vi "Aero_tunnel_monitor.vi"() -> ()   [LabVIEW 2011]
uses:
  Controls/Post_Process.ctl
  ADAM Client/Sub VIs/ADAM Controls/Update_scan_value.ctl
  Globals/Meas_global.vi
  <userlib>/LV-Link3/PolySubVIs/DtCreateAoutChan.vi
  <userlib>/LV-Link3/PolySubVIs/DtOLWriteSingle.vi
panel:
  in  "Display Graph?":bool
  in  "Menu Ring":u16(ring) items=["Lift", "Pitch", "Drag", "Side", "Yaw", "Roll"]
  in  "Samples":i32=1000
  out "Waveform Chart":dbl[](graph)
  in  "Output Roll":bool
  out "Roll":string="0.0 Nm"
  in  "Output Yaw":bool
  out "Yaw":string="0.0 Nm"
  in  "Output Pitch":bool
  out "Pitch":string="0.0 Nm"
  in  "Output SF":bool
  out "SF":string="0.0 N"
  in  "Output Drag":bool
  out "Drag":string="0.0 N"
  in  "Output Lift":bool
  out "Lift":string="0.0 N"
  in  "Balance Safey limits":T1(array[cluster])=[{"Max +ve Range"=80, "Max -ve Range"=80, "Axis"="Lift"}, {"Max +ve Range"=80, "Max -ve Range"=80, "Axis"="Pitch"}, {"Max +ve Range"=80, "Max -ve Range"=80, "Axis"="Drag"}, {"Max +ve Range"=80, "Max -ve Range"=80, "Axis"="Side-Force"}, {"Max +ve Range"=99, "Max -ve Range"=99, "Axis"="Yaw"}, {"Max +ve Range"=80, "Max -ve Range"=80, "Axis"="Roll"}] {"Max -ve Range" min=0 max=100; "Max +ve Range" min=0 max=100}
  out "Monitor Speed (Hz)":dbl=1765.7669969251795
  out "Belt slip warning":bool
  out "Road Status":string="???"
  in  "GotoYaw":bool
  in  "NewYawPos":dbl
  out "YAW POSITION":dbl
  out "Required WindSpeedRatio":dbl
  out "ROAD SPEED m/s":dbl
  in  "BL Fan1":i32
  in  "BL Fan2":i32
  in  "Stop drive":bool
  in  "Start Drive":bool
  in  "Synch to Wind":bool
  out "Road Info":string="???"
  in  "stop":bool
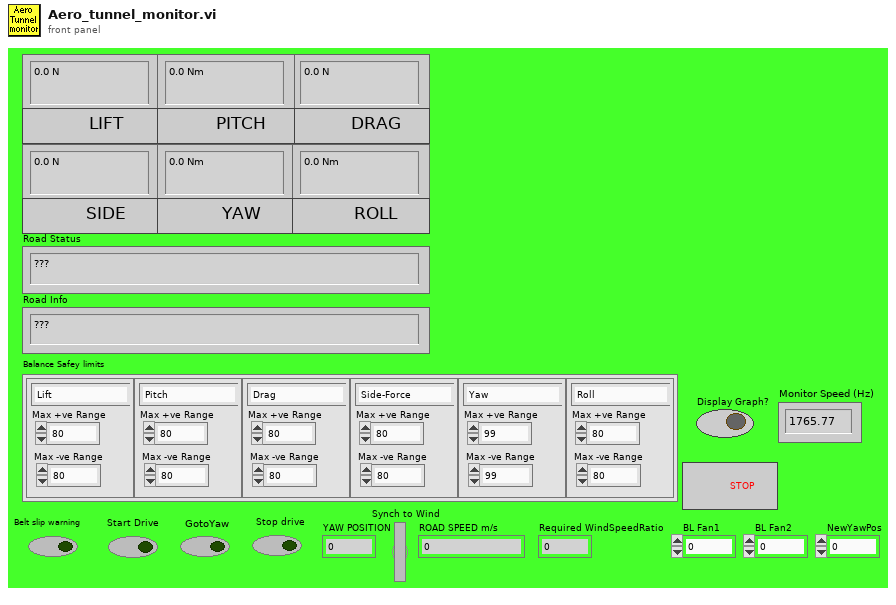
[diagram p1: front panel]
types:
  T1 = cluster{"Max +ve Range":i32, "Max -ve Range":i32, "Axis":string}[]
  T2 = typedef "Post_Process.ctl" = enum16{"Take New Data", "Post Process Raw Data File"}
  T3 = typedef "Update_scan_value.ctl" = cluster{"Channel Name":string, "New Value":dbl}
  T4 = cluster{"Max +ve Range":i32, "Max -ve Range":i32, "Axis":string}
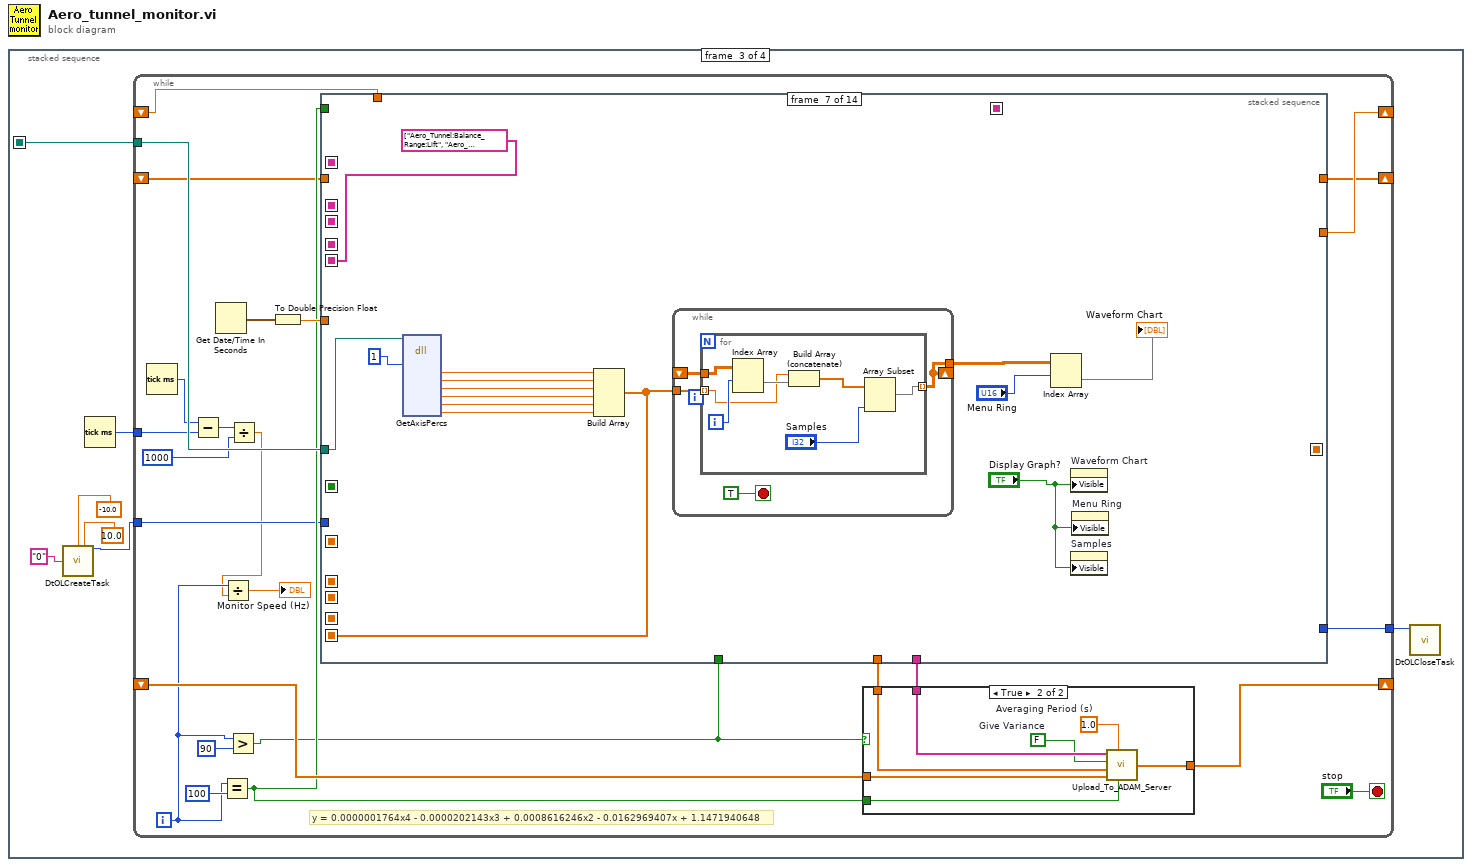
[diagram p0: block diagram]
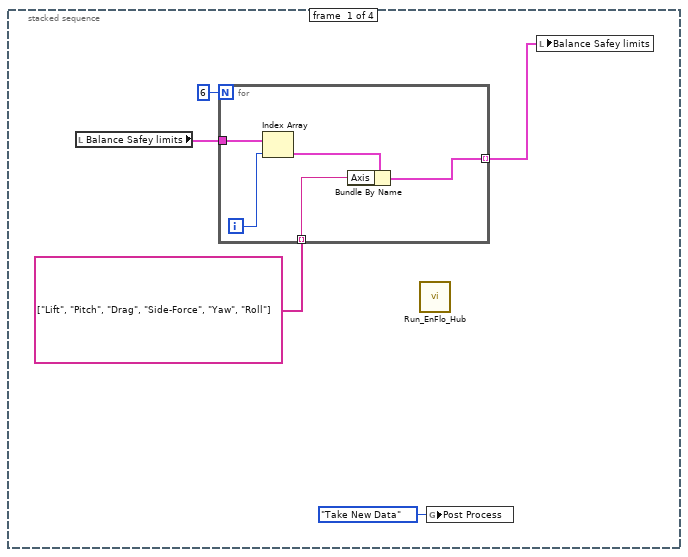
[diagram p2: hidden frame]
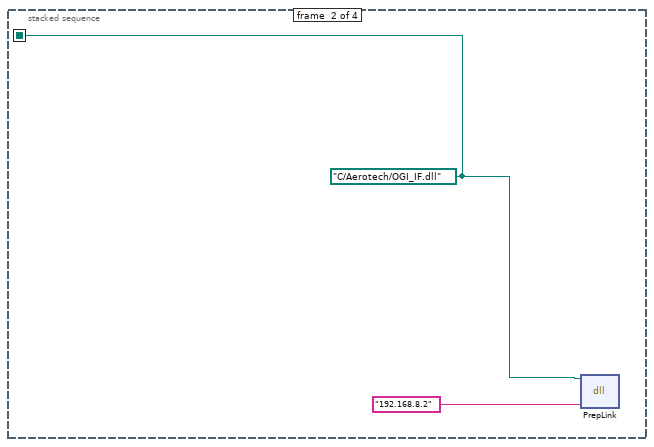
[diagram p3: hidden frame]
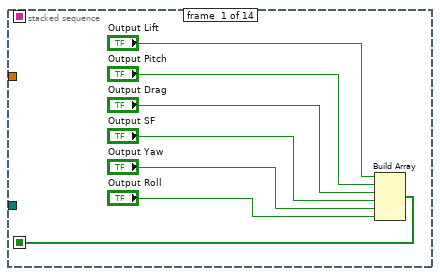
[diagram p5: hidden frame]
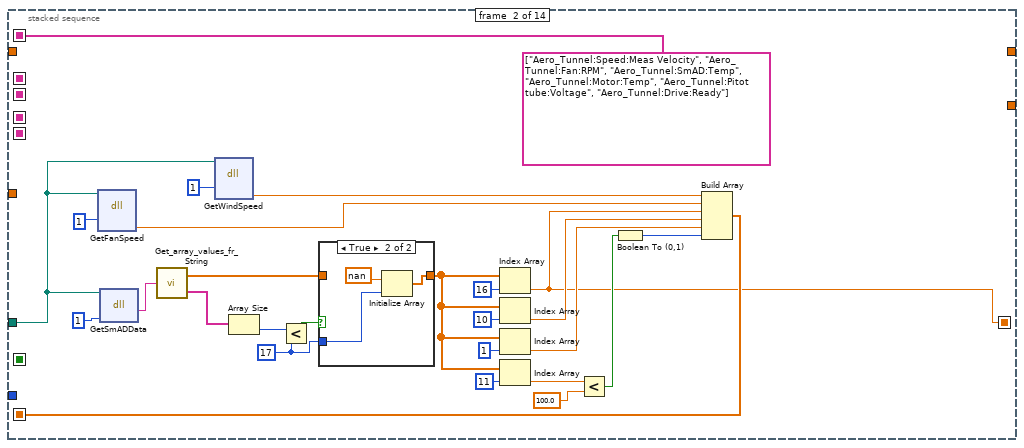
[diagram p6: hidden frame]
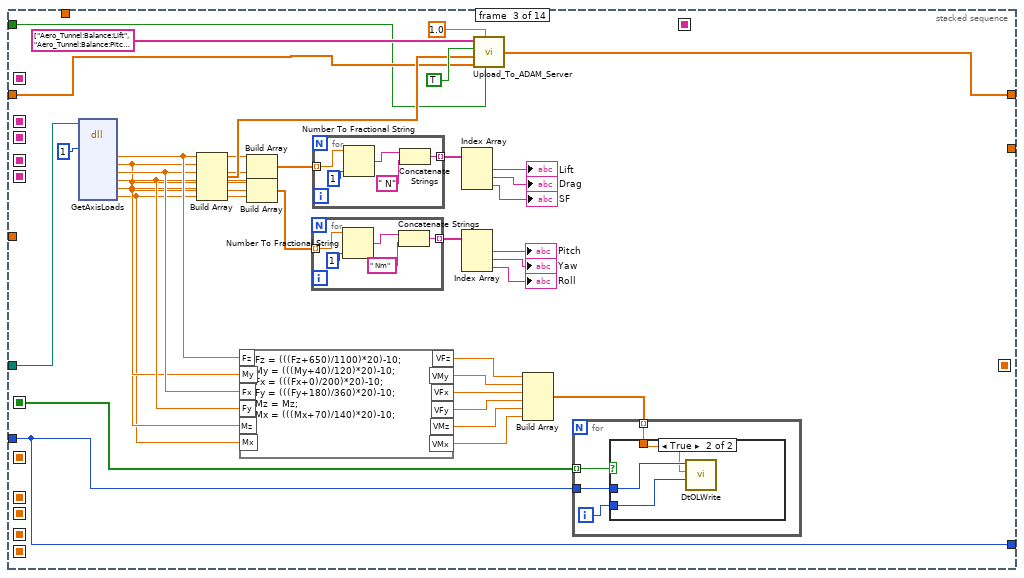
[diagram p8: hidden frame]
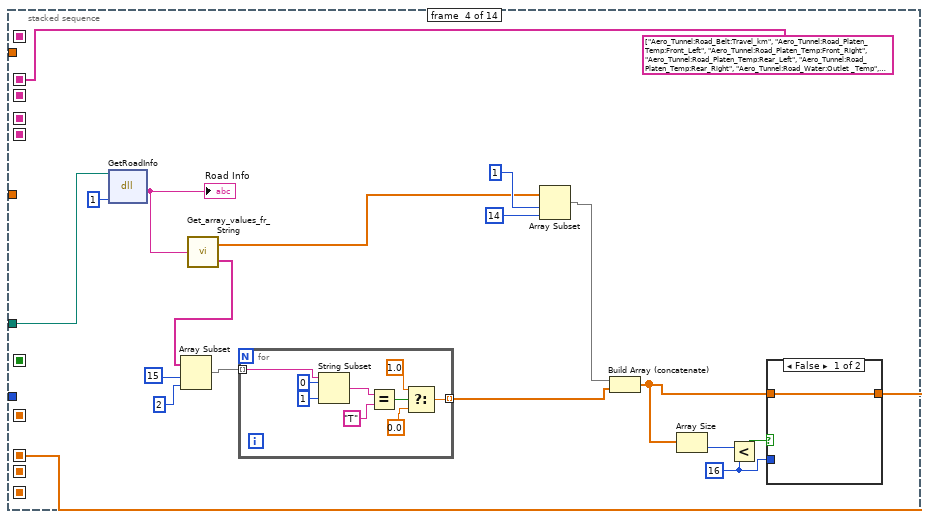
[diagram p10: hidden frame]
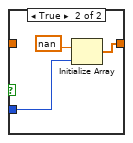
[diagram p11: hidden frame]
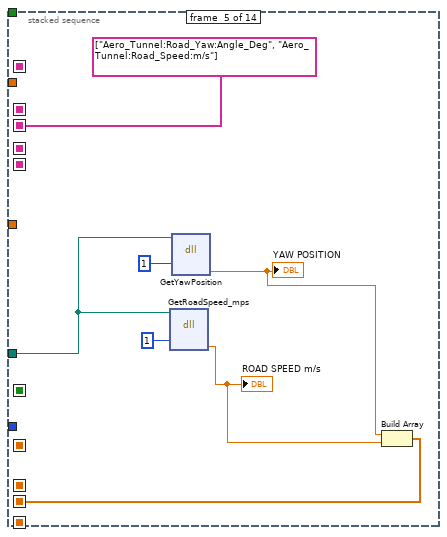
[diagram p12: hidden frame]
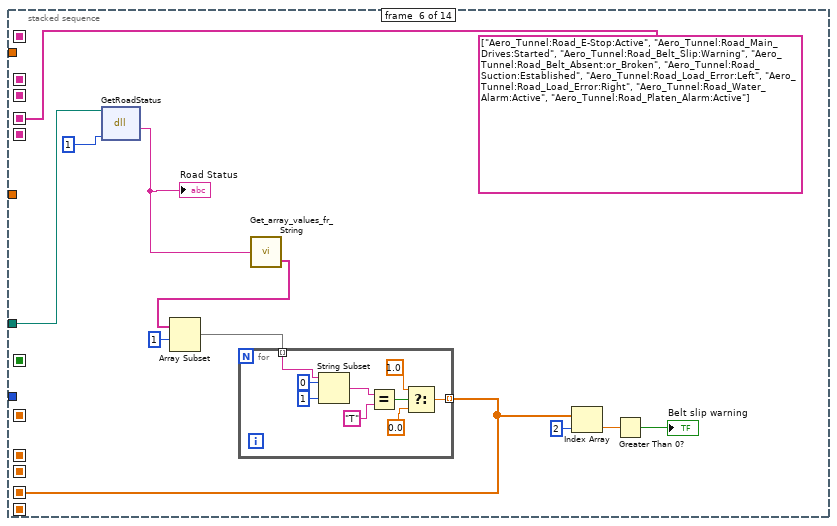
[diagram p13: hidden frame]
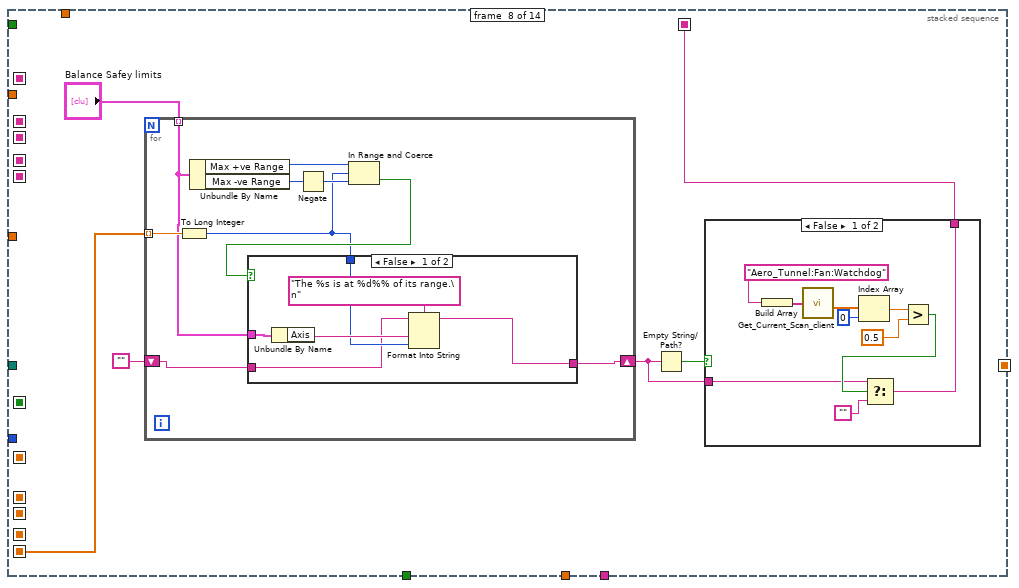
[diagram p14: hidden frame]
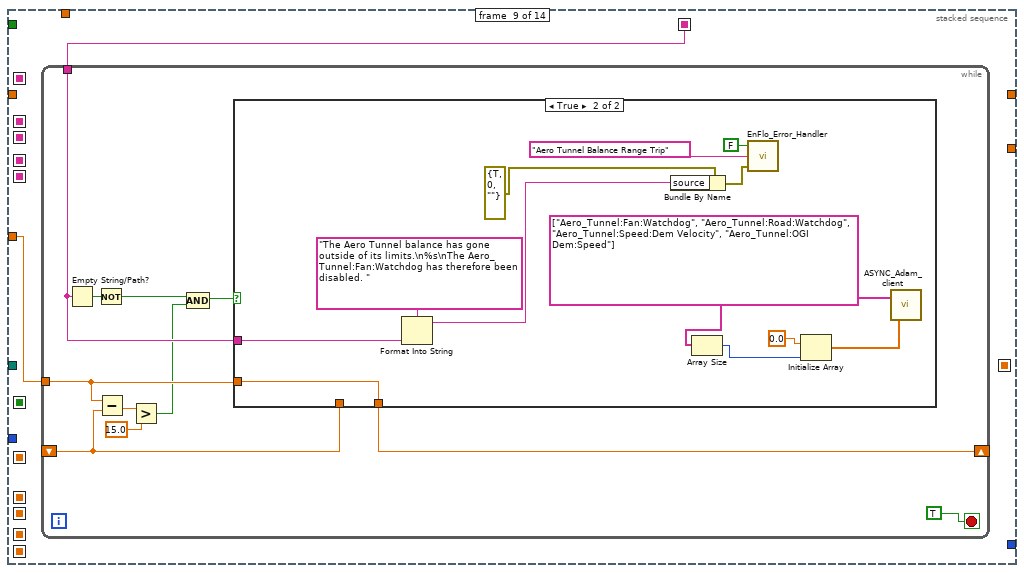
[diagram p17: hidden frame]
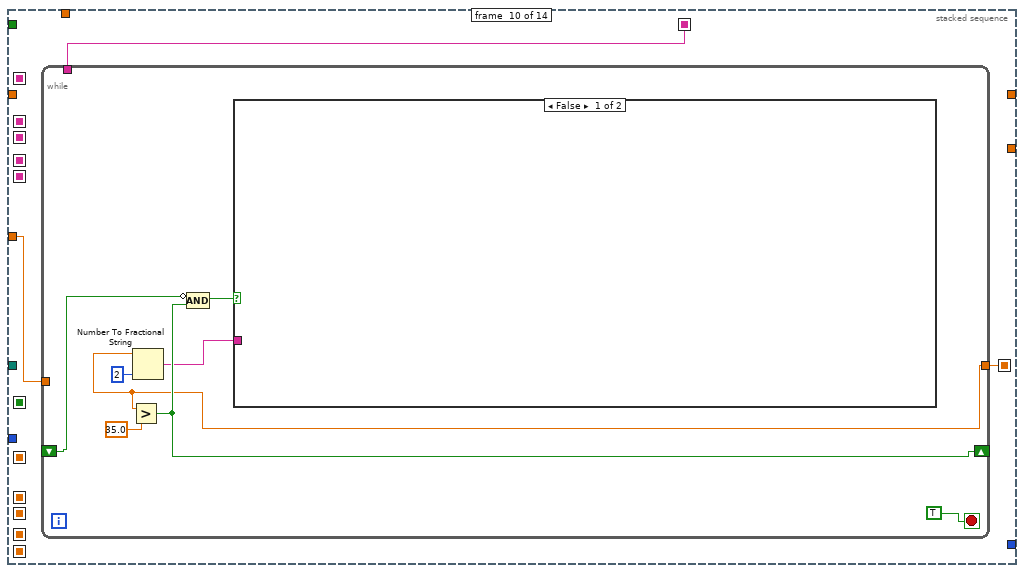
[diagram p19: hidden frame]
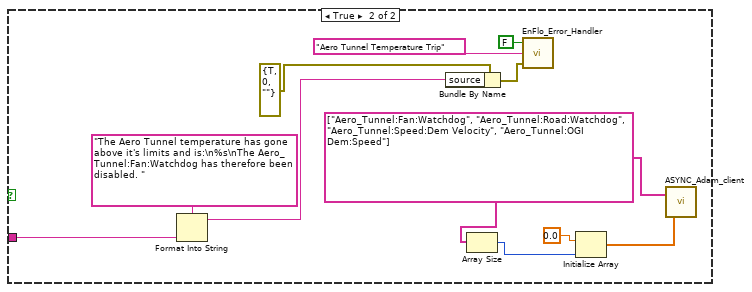
[diagram p20: hidden frame]
diagram:
  n1 = stacked-sequence {
    seq-local: [_ w11 _ _] -> [_ _ w19 w522]
    frame #0 {
      n2 = local read "Balance Safey limits"() -> (w4:T1)
      n3 = for {
        N: 6 -> [_]
        tunnel: w4 -> [w10]
        tunnel: [w7] -> w3 mode=indexing
        tunnel: string[] ["Lift", "Pitch", "Drag", "Side-Force", "Yaw", "Roll"] ("Channel Names") -> [w6] mode=indexing
        i -> [w9]
        n4 = Index Array(array=w10, index=w9) -> (element=w8:T4)
        n5 = Bundle By Name(cluster=w8, "Axis"=w6) -> (w7:T4)
      }
      n6 = call "Run_EnFlo_Hub.vi"() -> ()  [unwired: 8 in]
      n7 = global write "Meas_global.vi" "Post Process"(Post_Process."Take New Data" ("Post Process")) -> ()
      n8 = local write "Balance Safey limits"(w3) -> ()
    }
    frame #1 {
      w11 = path "C:/Aerotech/OGI_IF.dll" ("path in")
      n9 = dll-call lib="C:/Aerotech/Drivers/OGI_IF.dll" fn="PrepLink"(path in=w11, "IPAddress"="192.168.8.2") -> ()  [unwired: 2 in, 4 out]
    }
    frame #2 {
      n10 = call-poly <userlib>:"DtOLCreateTask.vi"("Range Min"=-10.0, "Range Max"=10.0, "Channel"="0" ("Channels")) -> ("Task out"=w14:i32)  [unwired: 10 in, 2 out]
      n11 = Tick Count (ms)() -> (millisecond timer value=w18:u32)
      n12 = while {
        shift-right: [w44] -> _
        shift-left: _ -> [w42]
        tunnel: w19 -> [w40]
        shift-right: [w35] -> _
        shift-left: _ -> [w38]
        tunnel: [w31] -> w13
        tunnel: w14 -> [w30]
        tunnel: w18 -> [w28]
        shift-right: [w20] -> _
        shift-left: _ -> [w21]
        i -> [w25]
        stop <- "stop" stop-if-true
        # "y = 0.0000001764x4 - 0.0000202143x3 + 0.0008616246x2 - 0.0162969407x + 1.1471940648"
        n13 = Tick Count (ms)() -> (millisecond timer value=w29:u32)
        n14 = Subtract(x=w29, y=w28) -> (x-y=w27:u32)
        n15 = Get Date/Time In Seconds() -> (seconds since 1Jan1904=w37:timestamp)
        n16 = Equal?(x=w25, y=100) -> (x = y?=w34:bool)
        n17 = Greater?(x=w25, y=90) -> (0:w22:bool)
        n18 = Divide(x=w27, y=u32 1000) -> (x/y=w24:dbl)
        n19 = Divide(x=w25, y=w24) -> (x/y=→"Monitor Speed (Hz)":dbl)
        n20 = To Double Precision Float(number=w37) -> (double precision float=w36:dbl)
        n21 = stacked-sequence {
          seq-local: [_ string[] ["Aero_Tunnel:Speed:Meas Velocity", "Aero_Tunnel:Fan:RPM", "Aero_Tunnel:SmAD:Temp", "Aero_Tunnel:Motor:Temp", "Aero_Tunnel:Pitot tube:Voltage", "Aero_Tunnel:Drive:Ready"] ("Channel Names") _ _ _ _ _ _ _ _ _ _ _ _] -> [_ _ _ _ _ _ _ _ _ _ w320 _ _ _]
          seq-local: [_ w75 _ _ _ _ _ _ _ _ _ _ _ _] -> [_ _ _ _ _ _ _ _ _ _ w319 _ _ _]
          seq-local: [_ _ _ w141 _ _ _ _ _ _ _ _ _ _] -> [_ _ _ _ _ _ _ _ _ _ w316 _ _ _]
          seq-local: [_ _ _ string[] ["Aero_Tunnel:Road_Belt:Travel_km", "Aero_Tunnel:Road_Platen_Temp:Front_Left", "Aero_Tunnel:Road_Platen_Temp:Front_Right", "Aero_Tunnel:Road_Platen_Temp:Rear_Left", "Aero_Tunnel:Road_Platen_Temp:Rear_Right", "Aero_Tunnel:Road_Water:Outlet _Temp", "Aero_Tunnel:Road_Water:Inlet _Temp", "Aero_Tunnel:Road_Suction:Front", "Aero_Tunnel:Road_Suction:Middle", "Aero_Tunnel:Road_Suction:Rear", "Aero_Tunnel:Road_BL_Suction:Primary", "Aero_Tunnel:Road_BL_Suction:Secondary", "Aero_Tunnel:Road_LoadCell:Left", "Aero_Tunnel:Road_LoadCell:Right", "Aero_Tunnel:Road_Water_High:Temp_Alarm", "Aero_Tunnel:Road_Platen_High:Temp_Alarm"] ("Channel Names") _ _ _ _ _ _ _ _ _ _] -> [_ _ _ _ _ _ _ _ _ _ w305 _ _ _]
          seq-local: [_ _ _ _ string[] ["Aero_Tunnel:Road_Yaw:Angle_Deg", "Aero_Tunnel:Road_Speed:m/s"] ("Channel Names") _ _ _ _ _ _ _ _ _] -> [_ _ _ _ _ _ _ _ _ _ w315 _ _ _]
          seq-local: [_ _ _ _ w172 _ _ _ _ _ _ _ _ _] -> [_ _ _ _ _ _ _ _ _ _ w314 _ _ _]
          seq-local: [_ _ _ _ _ string[] ["Aero_Tunnel:Road_E-Stop:Active", "Aero_Tunnel:Road_Main_Drives:Started", "Aero_Tunnel:Road_Belt_Slip:Warning", "Aero_Tunnel:Road_Belt_Absent:or_Broken", "Aero_Tunnel:Road_Suction:Established", "Aero_Tunnel:Road_Load_Error:Left", "Aero_Tunnel:Road_Load_Error:Right", "Aero_Tunnel:Road_Water_Alarm:Active", "Aero_Tunnel:Road_Platen_Alarm:Active"] ("Channel Names") _ _ _ _ _ _ _ _] -> [_ _ _ _ _ _ _ _ _ _ w310 _ _ _]
          seq-local: [_ _ _ _ _ w185 _ _ _ _ _ _ _ _] -> [_ _ _ _ _ _ _ _ _ _ w309 _ _ _]
          seq-local: [w59 _ _ _ _ _ _ _ _ _ _ _ _ _] -> [_ _ w115 _ _ _ _ _ _ _ _ _ _ _]
          seq-local: [_ _ _ _ _ _ string[] ["Aero_Tunnel:Balance_Range:Lift", "Aero_Tunnel:Balance_Range:Pitch", "Aero_Tunnel:Balance_Range:Drag", "Aero_Tunnel:Balance_Range:Side-Force", "Aero_Tunnel:Balance_Range:Yaw", "Aero_Tunnel:Balance_Range:Roll"] ("Channel Names") _ _ _ _ _ _ _] -> [_ _ _ _ _ _ _ _ _ _ w306 _ _ _]
          seq-local: [_ _ _ _ _ _ w203 _ _ _ _ _ _ _] -> [_ _ _ _ _ _ _ w228 _ _ w307 _ _ _]
          seq-local: [_ _ _ _ _ _ _ w224 _ _ _ _ _ _] -> [_ _ _ _ _ _ _ _ w258 w285 _ _ _ _]
          seq-local: [_ w60 _ _ _ _ _ _ _ _ _ _ _ _] -> [_ _ _ _ _ _ _ _ _ w283 _ _ _ _]
          tunnel: [_ _ _ _ _ _ _ _ _ _ w318 _ _ _] -> w43
          tunnel: [_ _ _ _ _ _ _ _ _ _ w317 _ _ _] -> w41
          tunnel: w40 -> [_ w67 w122 w157 w175 w188 w212 _ _ _ w308 w325 w438 w464]
          tunnel: w36 -> [_ _ _ _ _ _ _ _ w257 w284 _ w323 w437 _]
          tunnel: w38 -> [_ _ _ _ _ _ _ _ _ _ _ w322 _ _]
          tunnel: [_ _ _ _ _ _ _ _ _ _ _ w324 _ _] -> w35
          tunnel: w34 -> [_ _ w106 _ _ _ _ _ _ _ _ _ _ w465]
          tunnel: [_ _ w113 _ _ _ _ _ _ _ _ _ _ _] -> w31
          tunnel: w30 -> [_ _ w113 _ _ _ _ _ _ _ _ _ _ _]
          tunnel: w22 -> [_ _ _ _ _ _ _ _ _ _ _ w321 w436 _]
          tunnel: w21 -> [_ _ w108 _ _ _ _ _ _ _ _ _ _ _]
          tunnel: [_ _ w107 _ _ _ _ _ _ _ _ _ _ _] -> w20
          frame #0 {
            n22 = Build Array("Output Lift", "Output Pitch", "Output Drag", "Output SF", "Output Yaw", "Output Roll") -> (w59:bool[])
          }
          frame #1 {
            w61 = 17 ("y")
            n23 = dll-call lib="C:/Aerotech/Drivers/OGI_IF.dll" fn="GetFanSpeed"(path in=w67, "Enable"=1) -> ("FanSpeedinRPM"=w69:dbl)  [unwired: 3 in, 4 out]
            n24 = dll-call lib="C:/Aerotech/Drivers/OGI_IF.dll" fn="GetSmADData"(path in=w67, "Enable"=1) -> ("SmAD Data String"=w72:string)  [unwired: 2 in, 3 out]
            n25 = call "Get_array_values_fr_String.vi"("String Value"=w72) -> ("Numeric Array"=w62:dbl[], "String array"=w65:string[])
            n26 = dll-call lib="C:/Aerotech/Drivers/OGI_IF.dll" fn="GetWindSpeed"(path in=w67, "Enable"=1) -> ("Windspeed_M/s"=w68:dbl)  [unwired: 3 in, 4 out]
            n27 = Array Size(array=w65) -> (size(s)=w66:i32)
            n28 = Less?(x=w66, y=w61) -> (x < y?=w64:bool)
            n29 = case shown="True" w64 {
              tunnel: [w86 w89] -> w63
              tunnel: w62 -> [w86 _]
              tunnel: w61 -> [_ w87]
              frame False {
              }
              frame True {
                n30 = Initialize Array(nan, w87) -> (w89:dbl[])
              }
            }
            n31 = Index Array(array=w63, index=16) -> (element=w60:dbl)
            n32 = Index Array(array=w63, index=10) -> (element=w83:dbl)
            n33 = Index Array(array=w63, index=1) -> (element=w81:dbl)
            n34 = Index Array(array=w63, index=11) -> (element=w79:dbl)
            n35 = Less?(x=w79, y=100.0) -> (x < y?=w77:bool)
            n36 = Boolean To (0,1)(Boolean=w77) -> (0, 1=w76:i16)
            n37 = Build Array(w68, w69, w60, w83, w81, w76) -> (w75:dbl[])
          }
          frame #2 {
            n38 = dll-call lib="C:/Aerotech/Drivers/OGI_IF.dll" fn="GetAxisLoads"(path in=w122, "Enable"=1) -> ("Lift"=w105:dbl, "Pitch"=w97:dbl, "Drag"=w104:dbl, "side"=w103:dbl, "Yaw"=w96:dbl, "Roll"=w95:dbl)  [unwired: 3 in, 9 out]
            n39 = Build Array(w105, w97, w104, w103, w96, w95) -> (w109:dbl[])
            n40 = formula code="VFz = (((Fz+650)/1100)*20)-10;\nVMy = (((My+40)/120)*20)-10;\nVFx = (((Fx+0)/200)*20)-10;\nVFy = (((Fy+180)/360)*20)-10;\nVMz = Mz;\nVMx = (((Mx+70)/140)*20)-10;"("Fz"=w105, "My"=w97, "Fx"=w104, "Fy"=w103, "Mz"=w96, "Mx"=w95) -> ("VFz"=w121:dbl, "VMy"=w120:dbl, "VFx"=w119:dbl, "VFy"=w118:dbl, "VMz"=w117:dbl, "VMx"=w116:dbl)
            n41 = Build Array(w105, w104, w103) -> (w102:dbl[])
            n42 = Build Array(w97, w96, w95) -> (w94:dbl[])
            n43 = for {
              tunnel: w94 -> [w124] mode=indexing
              tunnel: [w128] -> w93 mode=indexing
              n44 = Number To Fractional String(number=w124, precision (6)=i16 1) -> (F-format string=w125:string)  [unwired: 2 in]
              n45 = Concatenate Strings(w125, " Nm" ("string")) -> (w128:string)
            }
            n46 = for {
              tunnel: w102 -> [w129] mode=indexing
              tunnel: [w133] -> w101 mode=indexing
              n47 = Number To Fractional String(number=w129, precision (6)=i16 1) -> (F-format string=w130:string)  [unwired: 2 in]
              n48 = Concatenate Strings(w130, " N" ("string")) -> (w133:string)
            }
            n49 = Index Array(array=w101) -> (element #1=→"Lift":string, element #2=→"Drag":string, element #3=→"SF":string)  [unwired: 3 in]
            n50 = Index Array(array=w93) -> (element #1=→"Pitch":string, element #2=→"Yaw":string, element #3=→"Roll":string)  [unwired: 3 in]
            n51 = call "Upload_To_ADAM_Server.vi"("First Loop"=w106, "Averaging Period (s)"=1.0, "Shift In"=w108, "Channel Values"=w109, "Give Variance"=TRUE, "Channel Names"=string[] ["Aero_Tunnel:Balance:Lift", "Aero_Tunnel:Balance:Pitch", "Aero_Tunnel:Balance:Drag", "Aero_Tunnel:Balance:Side-Force", "Aero_Tunnel:Balance:Yaw", "Aero_Tunnel:Balance:Roll"]) -> ("Shift Out"=w107:dbl[])
            n52 = Build Array(w121, w120, w119, w118, w117, w116) -> (w114:dbl[])
            n53 = for {
              tunnel: w113 -> [w137]
              tunnel: w115 -> [w136] mode=indexing
              tunnel: w114 -> [w135] mode=indexing
              i -> [w134]
              n54 = case shown="True" w136 {
                tunnel: w137 -> [_ w140]
                tunnel: w135 -> [_ w138]
                tunnel: w134 -> [_ w139]
                frame False {
                }
                frame True {
                  n55 = call-poly <userlib>:"DtOLWrite.vi"("Timeout"=w139, "Data In"=w138, "Task in"=w140) -> ()  [unwired: 7 in, 2 out]
                }
              }
            }
          }
          frame #3 {
            w144 = 16 ("y")
            n56 = dll-call lib="C:/Aerotech/Drivers/OGI_IF.dll" fn="GetRoadInfo"(path in=w157, "Enable"=1) -> ("Road Info"=w156:string)  [unwired: 3 in, 2 out]
            "Road Info" <- w156
            n57 = call "Get_array_values_fr_String.vi"("String Value"=w156) -> ("Numeric Array"=w143:dbl[], "String array"=w147:string[])
            n58 = Array Subset(array=w147, index=15, length=2) -> (w151:string[])
            n59 = for {
              tunnel: w151 -> [w169] mode=indexing
              tunnel: [w163] -> w150 mode=indexing
              n60 = String Subset(string=w169, offset (0)=0, length (rest)=1 ("length (rest)")) -> (substring=w168:string)
              n61 = Equal?(x=w168, y="T") -> (x = y?=w166:bool)
              n62 = Select(t=1.0, s=w166, f=0.0) -> (s? t:f=w163:dbl)
            }
            n63 = Array Subset(array=w143, index=1, length=14) -> (w149:dbl[])
            n64 = Build Array (concatenate)(w149, w150) -> (w142:dbl[])
            n65 = Array Size(array=w142) -> (size(s)=w146:i32)
            n66 = Less?(x=w146, y=w144) -> (x < y?=w145:bool)
            n67 = case shown="False" w145 {
              tunnel: [w159 w162] -> w141
              tunnel: w142 -> [w159 _]
              tunnel: w144 -> [_ w160]
              frame False {
              }
              frame True {
                n68 = Initialize Array(nan, w160) -> (w162:dbl[])
              }
            }
          }
          frame #4 {
            n69 = dll-call lib="C:/Aerotech/Drivers/OGI_IF.dll" fn="GetRoadSpeed_mps"(path in=w175, "Enable"=1) -> ("RoadSpeed_mps"=w173:dbl)  [unwired: 3 in, 4 out]
            "ROAD SPEED m/s" <- w173
            n70 = dll-call lib="C:/Aerotech/Drivers/OGI_IF.dll" fn="GetYawPosition"(path in=w175, "Enable"=1) -> ("Yaw Position"=w174:dbl)  [unwired: 3 in, 4 out]
            "YAW POSITION" <- w174
            n71 = Build Array(w174, w173) -> (w172:dbl[])
          }
          frame #5 {
            n72 = dll-call lib="C:/Aerotech/Drivers/OGI_IF.dll" fn="GetRoadStatus"(path in=w188, "Enable"=1) -> ("Road Status"=w187:string)  [unwired: 3 in, 2 out]
            "Road Status" <- w187
            n73 = call "Get_array_values_fr_String.vi"("String Value"=w187) -> ("String array"=w181:string[])  [unwired: 1 out]
            n74 = Array Subset(array=w181, index=1) -> (w179:string[])  [unwired: 1 in]
            n75 = for {
              tunnel: [w191] -> w185 mode=indexing
              tunnel: w179 -> [w190] mode=indexing
              n76 = String Subset(string=w190, offset (0)=0, length (rest)=1 ("length (rest)")) -> (substring=w196:string)
              n77 = Equal?(x=w196, y="T") -> (x = y?=w194:bool)
              n78 = Select(t=1.0, s=w194, f=0.0) -> (s? t:f=w191:dbl)
            }
            n79 = Index Array(array=w185, index=2) -> (element=w183:dbl)
            n80 = Greater Than 0?(x=w183) -> (x > 0?=→"Belt slip warning":bool)
          }
          frame #6 {
            n81 = dll-call lib="C:/Aerotech/Drivers/OGI_IF.dll" fn="GetAxisPercs"(path in=w212, "Enable"=1) -> ("Lift"=w210:dbl, "Pitch"=w209:dbl, "Drag"=w208:dbl, "side"=w207:dbl, "Yaw"=w206:dbl, "Roll"=w205:dbl)  [unwired: 3 in, 9 out]
            n82 = Build Array(w210, w209, w208, w207, w206, w205) -> (w203:dbl[])
            n83 = while {
              shift-right: [w214] -> _
              shift-left: _ -> [w216]
              tunnel: w203 -> [w215]
              tunnel: [w214] -> w202
              stop <- TRUE stop-if-true
              n84 = for {
                tunnel: w216 -> [w219]
                tunnel: w215 -> [w217] mode=indexing
                tunnel: [w222] -> w214 mode=indexing
                i -> [w220]
                n85 = Index Array(array=w219, index (row)=w220) -> (element=w218:dbl[])  [unwired: 1 in]
                n86 = Build Array (concatenate)(w217, w218) -> (w223:dbl[])
                n87 = Array Subset(array=w223, length="Samples") -> (w222:dbl[])  [unwired: 1 in]
              }
            }
            n88 = Index Array(array=w202, index (row)="Menu Ring") -> (element=→"Waveform Chart":dbl[])  [unwired: 1 in]
            n89 = property on="Waveform Chart" class="WFChart (strict)"("Visible"="Display Graph?") -> ()  [unwired: 2 in, 2 out]
            n90 = property on="Samples" class="DigNum (strict)"("Visible"="Display Graph?") -> ()  [unwired: 2 in, 2 out]
            n91 = property on="Menu Ring" class="Ring (strict)"("Visible"="Display Graph?") -> ()  [unwired: 2 in, 2 out]
          }
          frame #7 {
            n92 = for {
              tunnel: "Balance Safey limits" -> [w244] mode=indexing
              tunnel: w228 -> [w247] mode=indexing
              shift-right: [w241] -> w225
              shift-left: "" -> [w242]
              n93 = To Long Integer(number=w247) -> (32bit integer=w243:i32)
              n94 = Unbundle By Name(w244) -> ("Max +ve Range"=w249:i32, "Max -ve Range"=w248:i32)
              n95 = Negate(x=w248) -> (-x=w246:i32)
              n96 = In Range and Coerce(upper limit=w249, x=w243, lower limit=w246) -> (In Range?=w245:bool)  [unwired: 1 out]
              n97 = case shown="False" w245 {
                tunnel: w244 -> [w255 _]
                tunnel: w243 -> [w253 _]
                tunnel: w242 -> [w251 w256]
                tunnel: [w250 w256] -> w241
                frame False {
                  n98 = Unbundle By Name(w255) -> ("Axis"=w254:string)
                  n99 = Format Into String(format string="The %s is at %d%% of its range.\n", initial string=w251, w254, w253) -> (resulting string=w250:string)  [unwired: 1 in, 1 out]
                }
                frame True {
                }
              }
            }
            n100 = Empty String/Path?(string/path=w225) -> (empty?=w226:bool)
            n101 = case shown="False" w226 {
              tunnel: w225 -> [w232 w240]
              tunnel: [w230 w240] -> w224
              frame False {
                n102 = Build Array("Aero_Tunnel:Fan:Watchdog") -> (w239:string[])
                n103 = call "Get_Current_Scan_client.vi"("ADAM Ch Names"=w239) -> ("Numerical Values"=w237:dbl[])  [unwired: 1 in, 2 out]
                n104 = Index Array(array=w237, index=0) -> (element=w235:dbl)
                n105 = Greater?(x=w235, y=0.5) -> (0:w233:bool)
                n106 = Select(t=w232, s=w233, f="") -> (s? t:f=w230:string)
              }
              frame True {
              }
            }
          }
          frame #8 {
            n107 = while {
              tunnel: w258 -> [w267]
              shift-right: [w264] -> _
              shift-left: _ -> [w262]
              tunnel: w257 -> [w263]
              stop <- TRUE stop-if-true
              n108 = Empty String/Path?(string/path=w267) -> (empty?=w269:bool)
              n109 = Not(x=w269) -> (.not. x?=w265:bool)
              n110 = Subtract(x=w263, y=w262) -> (x-y=w261:dbl)
              n111 = Greater?(x=w261, y=15.0) -> (0:w259:bool)
              n112 = Compound Arithmetic op=AND(w265, w259) -> (w268:bool)
              n113 = case shown="True" w268 {
                tunnel: w267 -> [_ w276]
                tunnel: [w270 w275] -> w264
                tunnel: w263 -> [_ w275]
                tunnel: w262 -> [w270 _]
                frame False {
                }
                frame True {
                  w274 = string[] ["Aero_Tunnel:Fan:Watchdog", "Aero_Tunnel:Road:Watchdog", "Aero_Tunnel:Speed:Dem Velocity", "Aero_Tunnel:OGI Dem:Speed"] ("Channel Names")
                  n114 = Format Into String(format string="The Aero Tunnel balance has gone outside of its limits.\n%s\nThe Aero_Tunnel:Fan:Watchdog has therefore been disabled. ", w276) -> (resulting string=w277:string)  [unwired: 2 in, 1 out]
                  n115 = Bundle By Name(cluster=errorcluster {"status"=TRUE, "code"=0, "source"=""} ("error in (no error)"), "source"=w277) -> (w279:errorcluster)
                  n116 = Array Size(array=w274) -> (size(s)=w273:i32)
                  n117 = call "EnFlo_Error_Handler.vi"("error in (no error)"=w279, "Error Type"="Aero Tunnel Balance Range Trip", "Dialog Box (T)"=FALSE) -> ()  [unwired: 3 out]
                  n118 = Initialize Array(0.0, w273) -> (w271:dbl[])
                  n119 = call "ASYNC_Adam_client.vi"("Values"=w271, "Channel Names"=w274) -> ()  [unwired: 2 out]
                }
              }
            }
          }
          frame #9 {
            n120 = while {
              tunnel: w285 -> [_]
              shift-right: [w290] -> _
              shift-left: _ -> [w289]
              tunnel: w284 -> [_]
              tunnel: w283 -> [w287]
              stop <- TRUE stop-if-true
              n121 = Greater?(x=w287, y=35.0) -> (0:w290:bool)
              n122 = Number To Fractional String(number=w287, precision (6)=i16 2) -> (F-format string=w286:string)  [unwired: 2 in]
              n123 = Compound Arithmetic op=AND(invert w289, w290) -> (w293:bool)
              n124 = case shown="False" w293 {
                tunnel: w286 -> [_ w298]
                frame False {
                }
                frame True {
                  w297 = string[] ["Aero_Tunnel:Fan:Watchdog", "Aero_Tunnel:Road:Watchdog", "Aero_Tunnel:Speed:Dem Velocity", "Aero_Tunnel:OGI Dem:Speed"] ("Channel Names")
                  n125 = Format Into String(format string="The Aero Tunnel temperature has gone above it's limits and is:\n%s\nThe Aero_Tunnel:Fan:Watchdog has therefore been disabled. ", w298) -> (resulting string=w299:string)  [unwired: 2 in, 1 out]
                  n126 = Bundle By Name(cluster=errorcluster {"status"=TRUE, "code"=0, "source"=""} ("error in (no error)"), "source"=w299) -> (w301:errorcluster)
                  n127 = Array Size(array=w297) -> (size(s)=w296:i32)
                  n128 = call "EnFlo_Error_Handler.vi"("error in (no error)"=w301, "Error Type"="Aero Tunnel Temperature Trip", "Dialog Box (T)"=FALSE) -> ()  [unwired: 3 out]
                  n129 = Initialize Array(0.0, w296) -> (w294:dbl[])
                  n130 = call "ASYNC_Adam_client.vi"("Values"=w294, "Channel Names"=w297) -> ()  [unwired: 2 out]
                }
              }
            }
          }
          frame #10 {
            n131 = Build Array (concatenate)(w319, w316, w314, w309, w307) -> (w318:dbl[])
            n132 = Build Array (concatenate)(w320, w305, w315, w310, w306) -> (w317:string[])
            n133 = Boolean To (0,1)(Boolean="GotoYaw") -> (0, 1=w313:i16)
            n134 = dll-call lib="C:/Aerotech/Drivers/OGI_IF.dll" fn="GotoYawPosition"(path in=w308, "Enable"=w313, "NewYawPos"="NewYawPos") -> ()  [unwired: 3 in, 4 out]
          }
          frame #11 {
            n135 = Subtract(x=w323, y=w322) -> (x-y=w328:dbl)
            n136 = Greater?(x=w328, y=0.5) -> (0:w326:bool)
            n137 = case shown="True" w326 {
              tunnel: w325 -> [_ w332]
              tunnel: [w329 w331] -> w324
              tunnel: w323 -> [_ w331]
              tunnel: w322 -> [w329 _]
              tunnel: w321 -> [_ w330]
              frame False {
              }
              frame True {
                # "Tweak"
                # "Speed"
                # "Tweak"
                # "Speed"
                n138 = stacked-sequence {
                  seq-local: [_ w346 _ _ _ _ _] -> [_ _ _ w386 w400 _ w423]
                  seq-local: [_ w337 _ _ _ _ _] -> [_ _ _ w385 w397 _ _]
                  seq-local: [_ w344 _ _ _ _ _] -> [_ _ _ _ _ w412 _]
                  seq-local: [_ w340 _ _ _ _ _] -> [_ _ _ _ _ _ w425]
                  seq-local: [_ w338 _ _ _ _ _] -> [_ _ _ _ w398 _ _]
                  seq-local: [_ w336 _ _ _ _ _] -> [_ _ _ _ w396 _ _]
                  seq-local: [string[] ["Aero_Tunnel:OGI Dem:Speed", "Froude:NPL:Atmos_Press", "Aero_Tunnel:Motor:Enable", "Aero_Tunnel:Speed:Calib Tweak", "Aero_Tunnel:Upper:Temp", "Aero_Tunnel:Lower:Temp", "Aero_Tunnel:SmAD:Temp", "Aero_Tunnel:Fan:Watchdog"] ("appended array") _ _ _ _ _ _] -> [_ w335 _ _ _ _ _]
                  seq-local: [_ w334 _ _ _ _ _] -> [_ _ w370 _ _ _ _]
                  tunnel: w332 -> [_ w348 _ w384 w399 w411 w426]
                  tunnel: w330 -> [_ _ _ _ _ _ w421]
                  frame #0 {
                  }
                  frame #1 {
                    n139 = call "Get_Current_Scan_client.vi"("ADAM Ch Names"=w335) -> ("Numerical Values"=w334:dbl[])  [unwired: 1 in, 2 out]
                    n140 = Index Array(array=w334, index=0) -> (element=w346:dbl)
                    n141 = Index Array(array=w334, index=3) -> (element=w338:dbl)
                    n142 = Index Array(array=w334, index=1) -> (element=w344:dbl)
                    n143 = while {
                      tunnel: w348 -> [w356]
                      tunnel: w346 -> [w355]
                      shift-right: [w355] -> _
                      shift-left: _ -> [w354]
                      shift-right: [w351] -> _
                      shift-left: _ -> [w352]
                      tunnel: w338 -> [w351]
                      tunnel: [w350] -> w337
                      tunnel: [w349] -> w336
                      stop <- TRUE stop-if-true
                      n144 = Not Equal?(x=w355, y=w354) -> (x != y?=w350:bool)
                      n145 = Not Equal?(x=w351, y=w352) -> (x != y?=w349:bool)
                      n146 = case shown="True" w350 {
                        tunnel: w356 -> [_ w357]
                        tunnel: w355 -> [_ w358]
                        frame False {
                        }
                        frame True {
                          n147 = Greater?(x=w358, y=0.2) -> (0:w359:bool)
                          n148 = Boolean To (0,1)(Boolean=w359) -> (0, 1=w362:i16)
                          n149 = dll-call lib="C:/Aerotech/Drivers/OGI_IF.dll" fn="SetFanSystemState"(path in=w357, "Enable"=1, "Fan ONOFF"=w362) -> ()  [unwired: 3 in, 4 out]
                        }
                      }
                    }
                    n150 = Index Array(array=w334, index=2) -> (element=w342:dbl)
                    n151 = Greater?(x=w342, y=0.5) -> (0:w340:bool)
                  }
                  frame #2 {
                    n152 = Index Array(array=w370, index=7) -> (element=w368:dbl)
                    n153 = Array Subset(array=w370, index=4, length=3) -> (w372:dbl[])
                    n154 = Array Max & Min(array=w372) -> (max value=w363:dbl)  [unwired: 3 out]
                    n155 = Greater?(x=w368, y=0.5) -> (0:w365:bool)
                    n156 = Greater?(x=w363, y=35.0) -> (0:w366:bool)
                    n157 = And(x=w366, y=w365) -> (x .and. y?=w364:bool)
                    n158 = case shown="True" w364 {
                      tunnel: w363 -> [_ w377]
                      frame False {
                      }
                      frame True {
                        n159 = Format Into String(format string="Aero Tunnel temp is %.1f. The Aero_Tunnel:Fan:Watchdog has therefore been disabled. ", w377) -> (resulting string=w375:string)  [unwired: 2 in, 1 out]
                        n160 = Bundle By Name(cluster=errorcluster {"status"=TRUE, "code"=0, "source"=""} ("error in (no error)"), "source"=w375) -> (w378:errorcluster)
                        n161 = call "EnFlo_Error_Handler.vi"("error in (no error)"=w378, "Error Type"="Aero Tunnel over temp", "Dialog Box (T)"=FALSE) -> ()  [unwired: 3 out]
                        n162 = call "ASYNC_Adam_client.vi"("Values"=dbl[] [0.0, 0.0], "Channel Names"=string[] ["Aero_Tunnel:Fan:Watchdog", "Aero_Tunnel:Road:Watchdog"]) -> ()  [unwired: 2 out]
                      }
                    }
                  }
                  frame #3 {
                    n163 = case shown="True" w385 {
                      tunnel: w386 -> [_ w393]
                      tunnel: w384 -> [_ w394]
                      frame False {
                      }
                      frame True {
                        n164 = call "Polynomial_convert.vi"("Calib constants"=dbl[] [1.1471940648, -0.0162969407, 0.0008616246, -2.02143e-05, 1.764e-07], "Voltage"=w393) -> ("Eng Values"=w390:dbl)  [unwired: 4 in]
                        n165 = In Range and Coerce(upper limit=1.12, x=w390, lower limit=0.88) -> (coerced(x)=w387:dbl)  [unwired: 1 out]
                        "Required WindSpeedRatio" <- w387
                        n166 = dll-call lib="C:/Aerotech/Drivers/OGI_IF.dll" fn="SetWindSpeedRatio"(path in=w394, "Enable"=1 ("t"), "Required WindSpeedRatio"=w387) -> ()  [unwired: 4 in, 3 out]
                      }
                    }
                  }
                  frame #4 {
                    n167 = Or(x=w397, y=w396) -> (x .or. y?=w395:bool)
                    n168 = case shown="True" w395 {
                      tunnel: w400 -> [_ w405]
                      tunnel: w399 -> [_ w403]
                      tunnel: w398 -> [_ w406]
                      frame False {
                      }
                      frame True {
                        n169 = Divide(x=w406, y=100.0) -> (x/y=w408:dbl)
                        n170 = Increment(x=w408) -> (x+1=w409:dbl)
                        n171 = Multiply(x=w409, y=w405) -> (x*y=w404:dbl)
                        n172 = call "Polynomial_convert.vi"("Calib constants"=dbl[] [36.127, 22.861], "Voltage"=w404) -> ("Eng Values"=w402:dbl)  [unwired: 4 in]
                        n173 = dll-call lib="C:/Aerotech/Drivers/ATE_Surrey_WTCS.dll" fn="SetFanspeed"(path in=w403, "Enable"=1 ("t"), "NewFanSpeed"=w402) -> ()  [unwired: 3 in, 4 out]
                      }
                    }
                  }
                  frame #5 {
                    n174 = while {
                      shift-right: [w414] -> _
                      shift-left: _ -> [w417]
                      tunnel: w412 -> [w414]
                      tunnel: w411 -> [w415]
                      stop <- TRUE stop-if-true
                      n175 = Equal?(x=w414, y=w417) -> (x = y?=w416:bool)
                      n176 = case shown="True" w416 {
                        tunnel: w415 -> [_ w420]
                        tunnel: w414 -> [_ w418]
                        frame False {
                        }
                        frame True {
                          n177 = dll-call lib="C:/Aerotech/Drivers/OGI_IF.dll" fn="SetNewbaroPr_mB"(path in=w420, "Enable"=1, "NewPressure"=w418) -> ()  [unwired: 3 in, 4 out]
                        }
                      }
                    }
                  }
                  frame #6 {
                    n178 = Greater?(x=w423, y=0.1) -> (0:w422:bool)
                    n179 = while {
                      shift-right: [w431] -> _
                      shift-left: _ -> [w430]
                      tunnel: w425 -> [w431]
                      tunnel: w426 -> [w433]
                      tunnel: w422 -> [w429]
                      tunnel: w421 -> [w427]
                      stop <- TRUE stop-if-true
                      n180 = Compound Arithmetic op=AND(w431, invert w430, w429, w427) -> (w428:bool)
                      n181 = case shown="True" w428 {
                        tunnel: w433 -> [_ w435]
                        frame False {
                        }
                        frame True {
                          n182 = dll-call lib="C:/Aerotech/Drivers/OGI_IF.dll" fn="SetPitotZero"(path in=w435, "Enable"=1) -> ()  [unwired: 2 in, 4 out]
                        }
                      }
                    }
                  }
                }
              }
            }
          }
          frame #12 {
            n183 = while {
              tunnel: w438 -> [w446]
              tunnel: w437 -> [w445]
              tunnel: w436 -> [w444]
              shift-right: [w442] -> _
              shift-left: _ -> [w443]
              shift-right: [w440] -> _
              shift-left: _ -> [w439]
              stop <- TRUE stop-if-true
              # "Do every 15 seconds"
              n184 = Subtract(x=w445, y=w443) -> (x-y=w449:dbl)
              n185 = Greater?(x=w449, y=15.0) -> (0:w447:bool)
              n186 = case shown="True" w447 {
                tunnel: w446 -> [_ _]
                tunnel: [w451 w454] -> w442
                tunnel: w445 -> [_ w454]
                tunnel: w443 -> [w451 _]
                tunnel: w444 -> [_ _]
                tunnel: [w450 w453] -> w440
                tunnel: w439 -> [w450 w452]
                frame False {
                }
                frame True {
                  n187 = stacked-sequence {
                    tunnel: [w463] -> w453
                    tunnel: w452 -> [w462]
                    frame #0 {
                      n188 = Select(t=1.0, s=w462, f=0.0) -> (s? t:f=w456:dbl)
                      n189 = Not(x=w462) -> (.not. x?=w463:bool)
                      n190 = Bundle By Name(cluster=T3 {"Channel Name"="Aero_Tunnel:Server:Pulse", "New Value"=0.0} ("Update Scan Value Cluster"), "New Value"=w456) -> (w458:T3)
                      n191 = Build Array(w458) -> (w457:T3[])
                      n192 = call "Update_Current_Value_client.vi"("Don't Bother with check?"=TRUE, "Update array in"=w457) -> ()
                    }
                  }
                }
              }
            }
          }
          frame #13 {
            n193 = while {
              shift-right: [w476] -> _
              shift-left: _ -> [w478]
              tunnel: w465 -> [w477]
              tunnel: w464 -> [w474]
              shift-right: [w472] -> _
              shift-left: _ -> [w473]
              shift-right: [w470] -> _
              shift-left: _ -> [w471]
              shift-right: [w467] -> _
              shift-left: _ -> [w469]
              shift-right: [w466] -> _
              shift-left: _ -> [w468]
              stop <- TRUE stop-if-true
              n194 = stacked-sequence {
                tunnel: w478 -> [w484 _ _ _]
                tunnel: w477 -> [w482 w493 w502 w513]
                tunnel: ["Synch to Wind" _ _ _] -> w476
                tunnel: w474 -> [w479 w491 w500 w515]
                tunnel: w473 -> [_ w490 _ _]
                tunnel: [_ "Start Drive" _ _] -> w472
                tunnel: w471 -> [_ _ w499 _]
                tunnel: [_ _ "Stop drive" _] -> w470
                tunnel: w469 -> [_ _ _ w512]
                tunnel: w468 -> [_ _ _ w509]
                tunnel: [_ _ _ "BL Fan1"] -> w467
                tunnel: [_ _ _ "BL Fan2"] -> w466
                frame #0 {
                  n195 = Not Equal?(x="Synch to Wind", y=w484) -> (x != y?=w483:bool)
                  n196 = Or(x=w483, y=w482) -> (x .or. y?=w480:bool)
                  n197 = case shown="True" w480 {
                    tunnel: "Synch to Wind" -> [_ w486]
                    tunnel: w479 -> [_ w485]
                    frame False {
                    }
                    frame True {
                      n198 = Boolean To (0,1)(Boolean=w486) -> (0, 1=w487:i16)
                      n199 = dll-call lib="C:/Aerotech/Drivers/OGI_IF.dll" fn="RoadSyncToWind"(path in=w485, "Enable"=1, "SynchState"=w487) -> ()  [unwired: 3 in, 4 out]
                    }
                  }
                }
                frame #1 {
                  n200 = Not Equal?(x="Start Drive", y=w490) -> (x != y?=w494:bool)
                  n201 = Or(x=w494, y=w493) -> (x .or. y?=w492:bool)
                  n202 = case shown="True" w492 {
                    tunnel: "Start Drive" -> [_ w497]
                    tunnel: w491 -> [_ w495]
                    frame False {
                    }
                    frame True {
                      n203 = Boolean To (0,1)(Boolean=w497) -> (0, 1=w496:i16)
                      n204 = dll-call lib="C:/Aerotech/Drivers/OGI_IF.dll" fn="StartRoadDrive"(path in=w495, "Enable"=w496) -> ()  [unwired: 2 in, 4 out]
                    }
                  }
                }
                frame #2 {
                  n205 = Not Equal?(x="Stop drive", y=w499) -> (x != y?=w503:bool)
                  n206 = Or(x=w503, y=w502) -> (x .or. y?=w501:bool)
                  n207 = case shown="True" w501 {
                    tunnel: "Stop drive" -> [_ w506]
                    tunnel: w500 -> [_ w504]
                    frame False {
                    }
                    frame True {
                      n208 = Boolean To (0,1)(Boolean=w506) -> (0, 1=w505:i16)
                      n209 = dll-call lib="C:/Aerotech/Drivers/OGI_IF.dll" fn="RoadStop"(path in=w504, "Enable"=w505) -> ()  [unwired: 2 in, 4 out]
                    }
                  }
                }
                frame #3 {
                  n210 = Not Equal?(x=w509, y="BL Fan2") -> (x != y?=w510:bool)
                  n211 = Not Equal?(x="BL Fan1", y=w512) -> (x != y?=w511:bool)
                  n212 = Compound Arithmetic op=OR(w511, w510, w513) -> (w514:bool)
                  n213 = case shown="True" w514 {
                    tunnel: w515 -> [_ w517]
                    tunnel: "BL Fan1" -> [_ w519]
                    tunnel: "BL Fan2" -> [_ w518]
                    frame False {
                    }
                    frame True {
                      w516 = 1 ("BL Fan (1 or 2)")
                      n214 = dll-call lib="C:/Aerotech/Drivers/OGI_IF.dll" fn="SetBoundaryPerc"(path in=w517, "enable"=w516, "BL Fan (1 or 2)"=1, "New Percentage"=w519) -> ()  [unwired: 4 in, 4 out]
                      n215 = dll-call lib="C:/Aerotech/Drivers/OGI_IF.dll" fn="SetBoundaryPerc"(path in=w517, "enable"=w516, "BL Fan (1 or 2)"=2, "New Percentage"=w518) -> ()  [unwired: 4 in, 4 out]
                    }
                  }
                }
              }
            }
          }
        }
        n216 = case shown="True" w22 {
          tunnel: [w45 w52] -> w44
          tunnel: w43 -> [_ w51]
          tunnel: w42 -> [w45 w50]
          tunnel: w41 -> [_ w49]
          tunnel: w34 -> [_ w47]
          frame False {
          }
          frame True {
            w46 = FALSE  # Give Variance
            w48 = 1.0  # Averaging Period (s)
            n217 = call "Upload_To_ADAM_Server.vi"("First Loop"=w47, "Averaging Period (s)"=w48, "Shift In"=w50, "Channel Values"=w51, "Give Variance"=w46, "Channel Names"=w49) -> ("Shift Out"=w52:dbl[])
          }
        }
      }
      n218 = call <userlib>:"DtOLCloseTask.vi"("Task in"=w13) -> ()  [unwired: 10 in, 1 out]
    }
    frame #3 {
      n219 = dll-call lib="C:/Aerotech/Drivers/OGI_IF.dll" fn="CloseLink"(path in=w522) -> ()  [unwired: 2 in, 3 out]
    }
  }
